vi "TimerCalc.vi"(6 "Active":bool, 9 "ElapsedTime in":dbl, 10 "Timeout[s]":dbl, 11 "timeOfLastCall":timestamp) -> (1 "ElapsedTime out":dbl, 2 "Done":bool, 3 "now":timestamp)   [LabVIEW 2024]
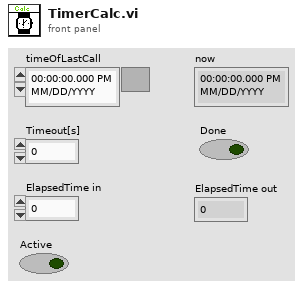
[diagram p1: front panel]
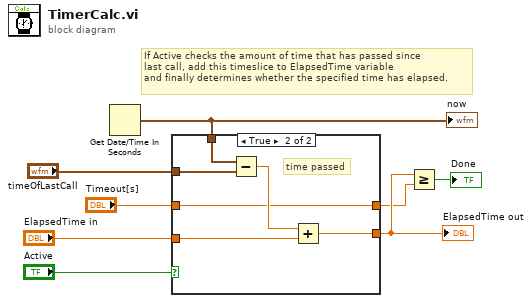
[diagram p0: block diagram]
diagram:
  # "If Active checks the amount of time that has passed since\nlast call, add this timeslice to ElapsedTime variable \nand finally determines whether the specified time has elapsed."
  n1 = Get Date/Time In Seconds() -> (seconds since 1Jan1904=w8:timestamp)
  "now" <- w8
  n2 = case shown="True" "Active" {
    tunnel: w8 -> [_ w16]
    tunnel: "ElapsedTime in" -> [w10 w15]
    tunnel: "Timeout[s]" -> [w9 w11]
    tunnel: "timeOfLastCall" -> [_ w13]
    tunnel: [w10 w12] -> w3
    tunnel: [w9 w11] -> w2
    frame False {
    }
    frame True {
      # "time passed"
      n3 = Subtract(x=w16, y=w13) -> (x-y=w14:dbl)
      n4 = Add(x=w14, y=w15) -> (x+y=w12:dbl)
    }
  }
  "ElapsedTime out" <- w3
  n5 = Greater Or Equal?(x=w3, y=w2) -> (x >= y?=→"Done":bool)
